vi "Recover from Lost Camera Connection.vi"() -> ()   [LabVIEW 2023]
doc: "The Recover from Lost Connection example acquires images continuously, and when there is an acquisition error (e.g. the camera is unplugged), the VI reconfigures the acquisition and resumes acquiring once the camera is available again."
uses:
  <vilib>/userdefined/High Color/IMAQdx.ctl
  <vilib>/vision/driver/NI_Vision_Acquisition_Software.lvlib
panel:
  in  "Invalid Session":T1
  in  "Camera Name":refnum<k21> caption="IMAQdx Session"
  out "Buffer Number":u32
  out "Acquiring":bool
  out "Image":T2(plugin-control)
  in  "Stop":bool
  # "Overview: Demonstrates how to restart an acquisition in the event that a camera is disconnected.\nRequirements: Vision Acquisition Software\nInstructions:\n1. Select the Camera Name.\n2. Run the VI\n3. While acquiring, disconnect the camera. Notice that the image does not update.\n4. Reconnect the camera. After reconfiguration, the camera acquires images again."
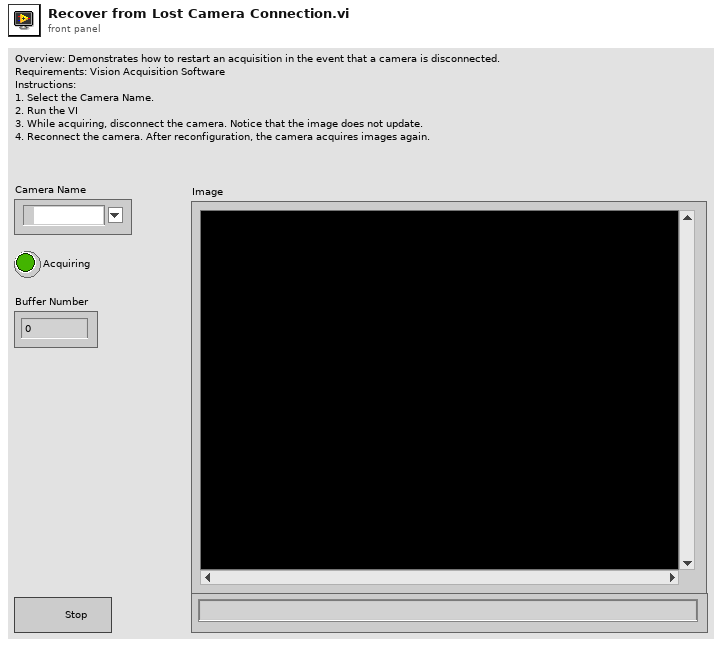
[diagram p1: front panel]
types:
  T1 = typedef "IMAQdx.ctl" = refnum<k21>
  T2 = typedef "IMAQ Image.ctl" = refnum<image>
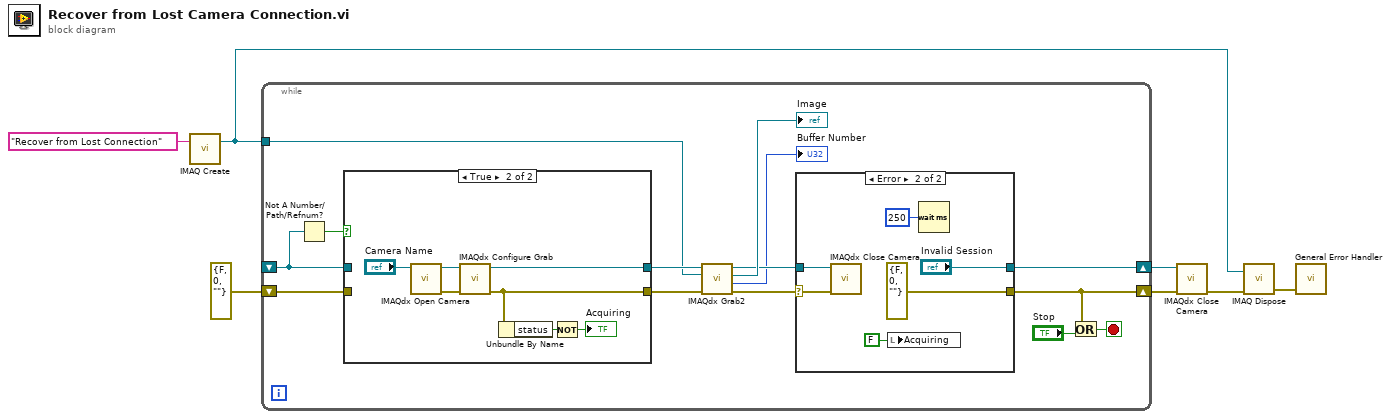
[diagram p0: block diagram]
diagram:
  n1 = call "IMAQ Create"("Image Name"="Recover from Lost Connection") -> ("New Image"=w1:T2)  [unwired: 3 in, 2 out]
  n2 = while {
    shift-right: [w13] -> w7
    shift-left: _ -> [w10]
    shift-right: [w9] -> w6
    shift-left: errorcluster {"status"=FALSE, "code"=0, "source"=""} ("error out") -> [w17]
    tunnel: w1 -> [w8]
    stop <- w21 stop-if-true
    n3 = Not A Number/Path/Refnum?(number/path/refnum=w10) -> (NaN/Path/Refnum?=w11:bool)
    n4 = case shown="True" w11 {
      tunnel: w10 -> [w31 _]
      tunnel: [w31 w36] -> w18
      tunnel: w17 -> [w30 _]
      tunnel: [w30 w35] -> w16
      frame False {
      }
      frame True {
        n5 = call <vilib>:"IMAQdx Open Camera.vi"("Session In"="Camera Name") -> ("error out"=w37:errorcluster, "Session Out"=w38:T1)  [unwired: 2 in, 7 out]
        n6 = call <vilib>:"IMAQdx Configure Grab.vi"("error in"=w37, "Session In"=w38) -> ("error out"=w35:errorcluster, "Session Out"=w36:T1)  [unwired: 1 in, 7 out]
        n7 = Unbundle By Name(w35) -> ("status"=w34:bool)
        n8 = Not(x=w34) -> (.not. x?=→"Acquiring":bool)
      }
    }
    n9 = call <vilib>:"IMAQdx Grab2.vi"("error in"=w16, "Image In"=w8, "Session In"=w18) -> ("error out"=w15:errorcluster, "Buffer Number Out"=→"Buffer Number":u32, "Image Out"=→"Image":T2, "Session Out"=w14:T1)  [unwired: 5 in]
    n10 = case shown="Error" w15 {
      selector: w15 -> [w23 w27]
      tunnel: [w23 errorcluster {"status"=FALSE, "code"=0, "source"=""} ("error IO")] -> w9
      tunnel: w14 -> [w22 w28]
      tunnel: [w22 "Invalid Session"] -> w13
      frame No Error {
      }
      frame Error {
        n11 = call <vilib>:"IMAQdx Close Camera.vi"("error in"=w27, "Session In"=w28) -> ()  [unwired: 10 out]
        n12 = local write "Acquiring"(FALSE ("Acquiring")) -> ()
        n13 = Wait (ms)(milliseconds to wait=u32 250) -> ()  [unwired: 1 out]
      }
    }
    n14 = Or(x=w9, y="Stop") -> (x .or. y?=w21:bool)
  }
  n15 = call <vilib>:"IMAQdx Close Camera.vi"("error in"=w6, "Session In"=w7) -> ("error out"=w3:errorcluster)  [unwired: 9 out]
  n16 = call "IMAQ Dispose"("Image"=w1, "error in (no error)"=w3) -> ("error out"=w2:errorcluster)  [unwired: 4 in]
  n17 = call <vilib>:"General Error Handler.vi"("error in (no error)"=w2) -> ()  [unwired: 2 in, 13 out]
